vi "Initialize Generate.vi"(8 "error in (no error)":errorcluster, 10 "PCL (usec)":u32, 11 "OnCompile Variables":T9={"XNET Settings"={"Database"="", "Cluster"="", "Port"="", "Baud rate [Bd]"=500000, "Termination"=1, "CAN I/O Mode"=0, "FD Baud rate [Bd]"=500000, "Priority"=100, "Use Legacy"=FALSE}, "Frames"=[], "986x Support"={"Enable"=FALSE, "RIO Device"="", "Bitfile"=path ""}, "Incoming Frames"=[]} {"Incoming Frames"."Protection Configurations"."CRC Channels"."Data Type" items=["Signed", "Unsigned", "IEEE Float"]; "XNET Settings"."CAN I/O Mode" items=["CAN 2.0", "CAN FD", "CAN FD+BRS"]; "XNET Settings"."Termination" items=["Off", "On"]; "Frames"."Protection Configurations"."CRC Channels"."Data Type" items=["Signed", "Unsigned", "IEEE Float"]}) -> (0 "error out":errorcluster, 3 "RT Configuration":T1={"Priority"=100, "CAN Session"="", "Frame Count"=0, "Frames"=[], "FPGA Session"=0, "Incoming Frame Session"="", "Incoming Session Invalid"=FALSE} {"Frames"."Protection Configurations"."CRC Channels"."Data Type" items=["Signed", "Unsigned", "IEEE Float"]})   [LabVIEW 2015, in "Protection and Counter Addon Engine.lvlib"]
uses:
  Protection and Counter Addon Engine.lvlib
  Shared/Types/Exported.OnCompile.ctl
  Shared/Types/XNET Settings.ctl
  SubModules/Frame Protection Support/Source/Shared/Types/Exported Frame Settings.ctl
  SubModules/Frame Protection Support/Source/Shared/Types/Exported Frame Type.ctl
  SubModules/Frame Protection Support/Source/Shared/Types/Exported Protection Settings.ctl
  SubModules/Frame Protection Support/Source/Shared/Types/Protection Type.ctl
  SubModules/Frame Protection Support/Source/Shared/Types/XNET Signal Configuration.ctl
  SubModules/Frame Protection Support/Source/Shared/Types/Exported Counter Settings.ctl
  SubModules/Frame Protection Support/Source/Shared/Types/Exported Event Trigger Type.ctl
  Shared/Types/986x.ctl
  Types/RT Async Engine Variables.ctl
  SubModules/Frame Protection Support/Source/Engine/Types/RT Frame Settings.ctl
  SubModules/Frame Protection Support/Source/Engine/Types/RT Protection Configuration.ctl
  <vilib>/xnet/xnet.llb/XNET Create Session (Frame Output Stream).vi
  SubModules/Frame Protection Support/Source/Shared/Protection and Counter Support Shared.lvlib
  SubModules/Frame Protection Support/Source/Engine/Protection and Counter Support Engine.lvlib
  <resource>/objmgr/xnet.rc
  Shared/Protection and Counter Addon Shared.lvlib
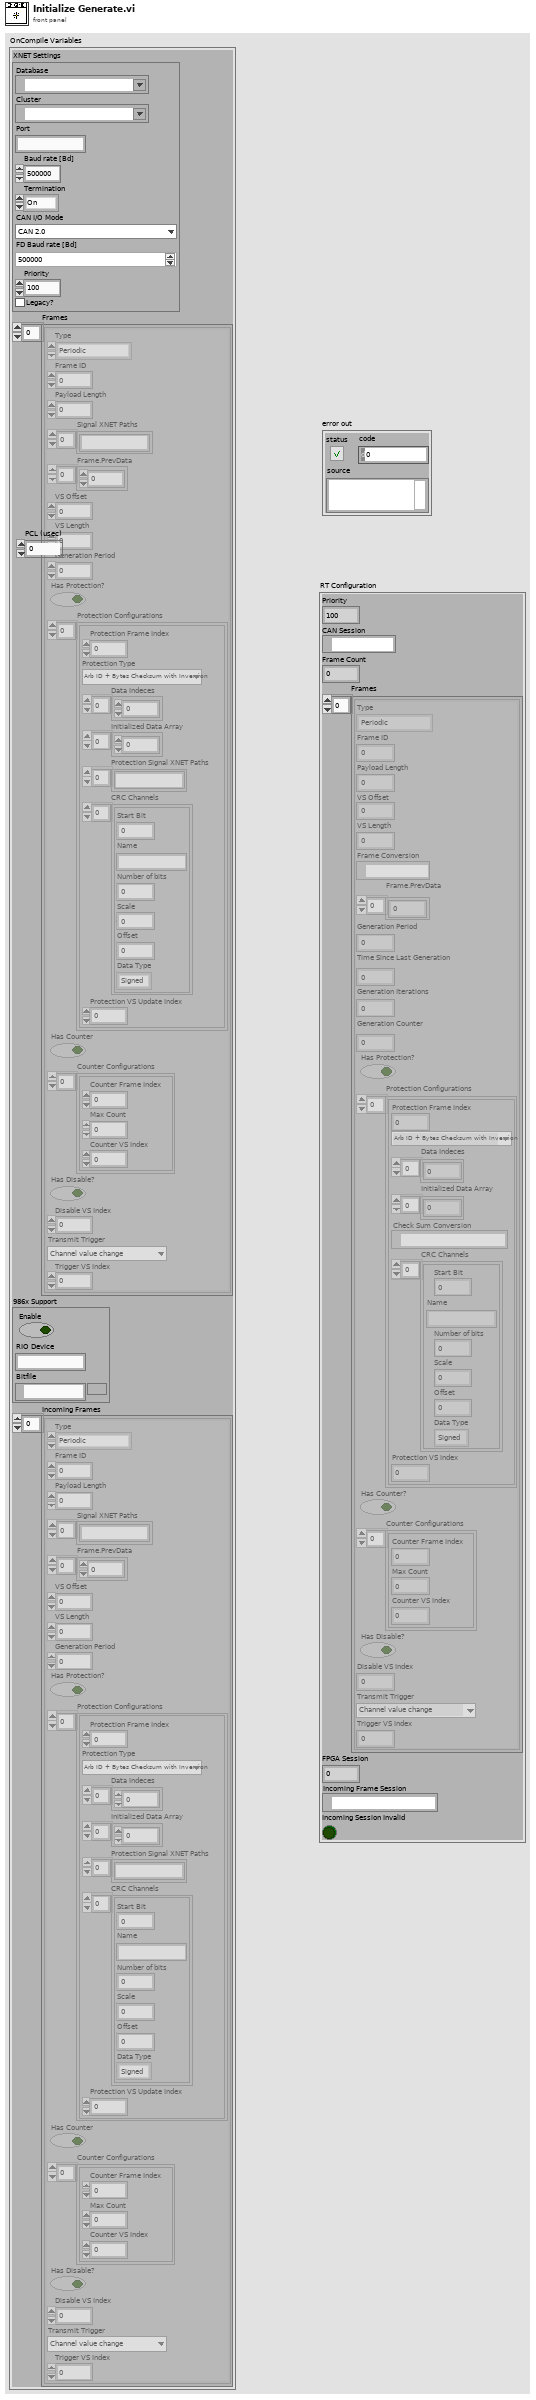
[diagram p1: front panel]
types:
  T1 = typedef "Protection and Counter Addon Engine.lvlib/RT Async Engine Variables.ctl" = cluster{"Priority":i32, "CAN Session":refnum<k21>, "Frame Count":i32, "Frames":T2[], "FPGA Session":u32, "Incoming Frame Session":refnum<k21>, "Incoming Session Invalid":bool}
  T2 = typedef "Protection and Counter Support Engine.lvlib/RT Frame Settings.ctl" = cluster{"Type":T3, "Frame ID":u32, "Payload Length":u32, "VS Offset":i32, "VS Length":i32, "Frame Conversion":refnum<k21>, "Frame.PrevData":dbl[], "Generation Period":u32, "Time Since Last Generation":u32, "Generation Iterations":u32, "Generation Counter":u32, "Has Protection?":bool, "Protection Configurations":T4[], "Has Counter?":bool, "Counter Configurations":T7[], "Has Disable?":bool, "Disable VS Index":i32, "Transmit Trigger":T8, "Trigger VS Index":i32}
  T3 = typedef "Protection and Counter Support Shared.lvlib/Exported Frame Type.ctl" = enum16{"Periodic", "Event", "Periodic/Event"}
  T4 = typedef "Protection and Counter Support Engine.lvlib/RT Protection Configuration.ctl" = cluster{"Protection Frame Index":i32, "Protection Type":T5, "Data Indeces":i32[], "Initialized Data Array":dbl[], "Check Sum Conversion":refnum<k21>, "CRC Channels":T6[], "Protection VS Index":i32}
  T5 = typedef "Protection and Counter Support Shared.lvlib/Protection Type.ctl" = enum16{"Arb ID + Bytes Checksum with Inversion", "Arb ID + Bytes CRC with Inversion", "Reversed Raw Signal Checksum with Inversion"}
  T6 = typedef "Protection and Counter Support Shared.lvlib/XNET Signal Configuration.ctl" = cluster{"Start Bit":i32, "Name":string, "Number of bits":i32, "Scale":dbl, "Offset":dbl, "Data Type":u32}
  T7 = typedef "Protection and Counter Support Shared.lvlib/Exported Counter Settings.ctl" = cluster{"Counter Frame Index":i32, "Max Count":dbl, "Counter VS Index":i32}
  T8 = typedef "Protection and Counter Support Shared.lvlib/Exported Event Trigger Type.ctl" = enum16{"Channel value change", "Trigger channel (not zero)", "Channel value change or trigger channel (not zero)", "Trigger channel (any value change)", "Channel value change or trigger channel (any value change)"}
  T9 = typedef "Protection and Counter Addon Shared.lvlib/Exported.OnCompile.ctl" = cluster{"XNET Settings":T10, "Frames":T11[], "986x Support":T13, "Incoming Frames":T11[]}
  T10 = typedef "Protection and Counter Addon Shared.lvlib/XNET Settings.ctl" = cluster{"Database":refnum<k21>, "Cluster":refnum<k21>, "Port":string, "Baud rate [Bd]":u64, "Termination":u32, "CAN I/O Mode":u32, "FD Baud rate [Bd]":u64, "Priority":i32, "Use Legacy":bool}
  T11 = typedef "Protection and Counter Support Shared.lvlib/Exported Frame Settings.ctl" = cluster{"Type":T3, "Frame ID":u32, "Payload Length":u32, "Signal XNET Paths":string[], "Frame.PrevData":dbl[], "VS Offset":i32, "VS Length":i32, "Generation Period":u32, "Has Protection?":bool, "Protection Configurations":T12[], "Has Counter":bool, "Counter Configurations":T7[], "Has Disable?":bool, "Disable VS Index":i32, "Transmit Trigger":T8, "Trigger VS Index":i32}
  T12 = typedef "Protection and Counter Support Shared.lvlib/Exported Protection Settings.ctl" = cluster{"Protection Frame Index":i32, "Protection Type":T5, "Data Indeces":i32[], "Initialized Data Array":dbl[], "Protection Signal XNET Paths":string[], "CRC Channels":T6[], "Protection VS Update Index":i32}
  T13 = typedef "Protection and Counter Addon Shared.lvlib/986x.ctl" = cluster{"Enable":bool, "RIO Device":string, "Bitfile":path}
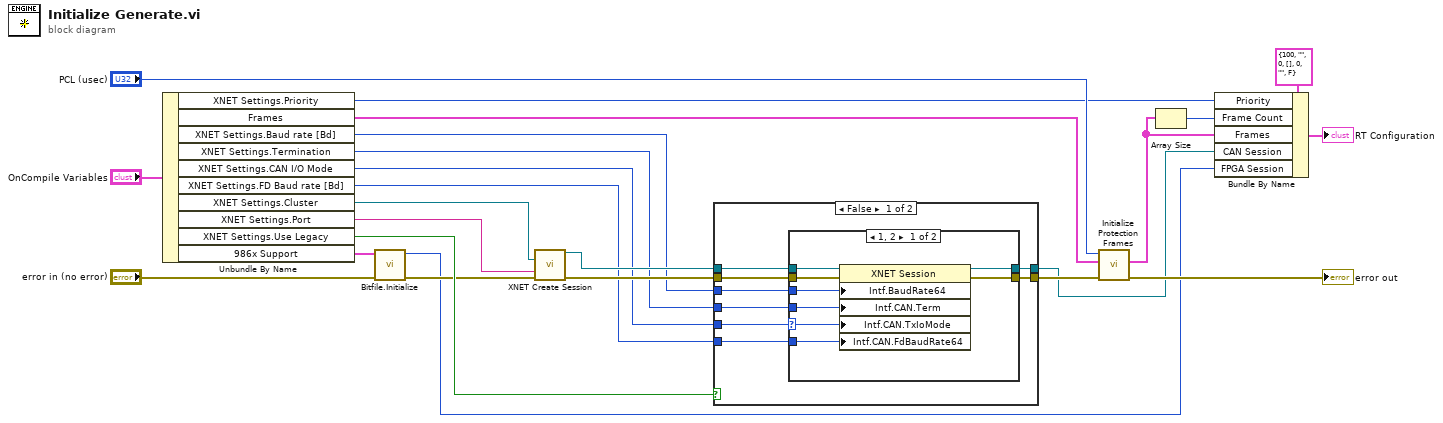
[diagram p0: block diagram]
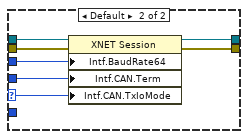
[diagram p2: hidden frame]
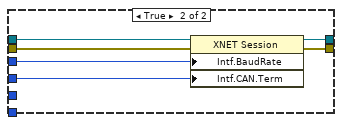
[diagram p3: hidden frame]
diagram:
  n1 = Unbundle By Name("OnCompile Variables") -> ("XNET Settings.Priority"=w8:i32, "Frames"=w23:T11[], "XNET Settings.Baud rate [Bd]"=w11:u64, "XNET Settings.Termination"=w12:u32, "XNET Settings.CAN I/O Mode"=w13:u32, "XNET Settings.FD Baud rate [Bd]"=w14:u64, "XNET Settings.Cluster"=w16:refnum<k21>, "XNET Settings.Port"=w15:string, "XNET Settings.Use Legacy"=w7:bool, "986x Support"=w4:T13)
  n2 = call "Bitfile.Initialize.vi"("error in (no error)"="error in (no error)", "FPGA Bitfile Settings"=w4) -> ("error out"=w5:errorcluster, "FPGA Session"=w3:u32)  [unwired: 8 in]
  n3 = call-poly <vilib>:"XNET Create Session.vi"("cluster (:memory:)"=w16, "interface"=w15, "error in (no error)"=w5) -> ("session out"=w18:refnum<k21>, "error out"=w19:errorcluster)  [unwired: 11 in]
  n4 = case shown="False" w7 {
    tunnel: w19 -> [w32 w53]
    tunnel: w18 -> [w31 w52]
    tunnel: [w30 w51] -> w17
    tunnel: w14 -> [w29 _]
    tunnel: w13 -> [w25 _]
    tunnel: w12 -> [w28 w48]
    tunnel: w11 -> [w27 w49]
    tunnel: [w26 w50] -> w1
    frame False {
      n5 = case shown="1, 2" w25 {
        selector: w25 -> [w33 w41]
        tunnel: w32 -> [w40 w47]
        tunnel: w31 -> [w39 w46]
        tunnel: [w38 w45] -> w30
        tunnel: w29 -> [w37 _]
        tunnel: w28 -> [w36 w44]
        tunnel: w27 -> [w35 w43]
        tunnel: [w34 w42] -> w26
        frame 1, 2 {
          n6 = property class="XNET Session"(reference=w39, error in=w40, "Intf.BaudRate64"=w35, "Intf.CAN.Term"=w36, "Intf.CAN.TxIoMode"=w33, "Intf.CAN.FdBaudRate64"=w37) -> (reference out=w34:refnum<k21>, error out=w38:errorcluster)
        }
        frame Default {
          n7 = property class="XNET Session"(reference=w46, error in=w47, "Intf.BaudRate64"=w43, "Intf.CAN.Term"=w44, "Intf.CAN.TxIoMode"=w41) -> (reference out=w42:refnum<k21>, error out=w45:errorcluster)
        }
      }
    }
    frame True {
      n8 = property class="XNET Session"(reference=w52, error in=w53, "Intf.BaudRate"=w49, "Intf.CAN.Term"=w48) -> (reference out=w50:refnum<k21>, error out=w51:errorcluster)
    }
  }
  n9 = call "Initialize Protection Frames.vi"("error in (no error)"=w17, "Frames"=w23, "PCL (usec)"="PCL (usec)") -> ("error out"=→"error out":errorcluster, "RT Frames"=w2:T2[])  [unwired: 7 in]
  n10 = Array Size(array=w2) -> (size(s)=w9:i32)
  n11 = Bundle By Name(cluster=T1 {"Priority"=100, "CAN Session"="", "Frame Count"=0, "Frames"=[], "FPGA Session"=0, "Incoming Frame Session"="", "Incoming Session Invalid"=FALSE} ("RT Configuration"), "Priority"=w8, "Frame Count"=w9, "Frames"=w2, "CAN Session"=w1, "FPGA Session"=w3) -> (→"RT Configuration":T1)
